vi "Num2NormString.vi"(1 "Number":u32) -> (0 "Normalized String Number":string)   [LabVIEW 2018]
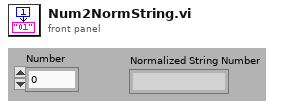
[diagram p1: front panel]
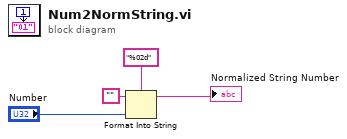
[diagram p0: block diagram]
diagram:
  n1 = Format Into String(format string="%02d" ("Substring"), initial string="", "Number") -> (resulting string=→"Normalized String Number":string)  [unwired: 1 in, 1 out]
